vi "TDMSCreateGraph.vi"(8 "error in (no error)":errorcluster, 9 "States":string, 10 "FitModel":string, 11 "TraceName":string="D:\\Vi\\Data\\Singapore\\170620\\data_145.tdms: 3") -> (0 "error out":errorcluster, 2 "F(z) Graph":cluster{"Data":dbl[], "Data":dbl[]}[](graph), 3 "z(t) Graph":cluster{"Data":dbl[], "Data":dbl[]}[](graph))   [LabVIEW 2018]
uses:
  <vilib>/Analysis/polynomials.llb/Unique Numbers and Multiplicity (DBL).vi
  <vilib>/Analysis/NI_AALPro.lvlib
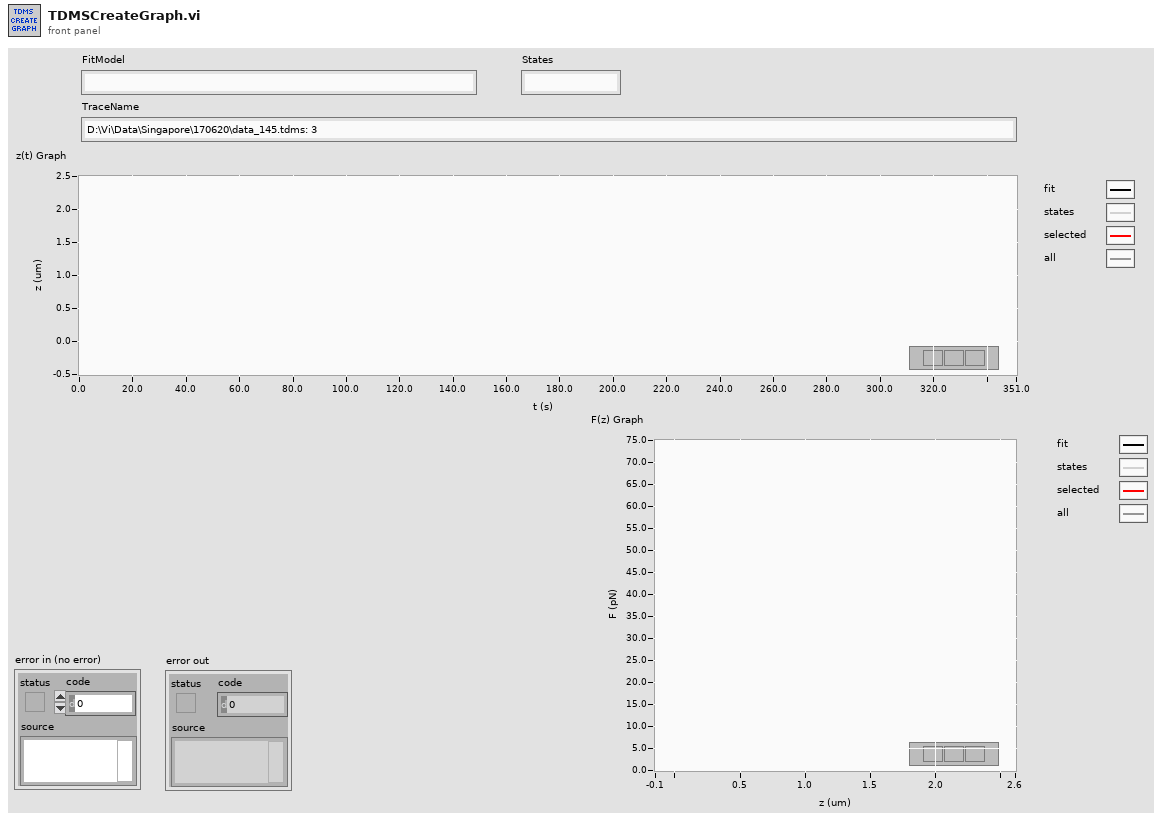
[diagram p1: front panel]
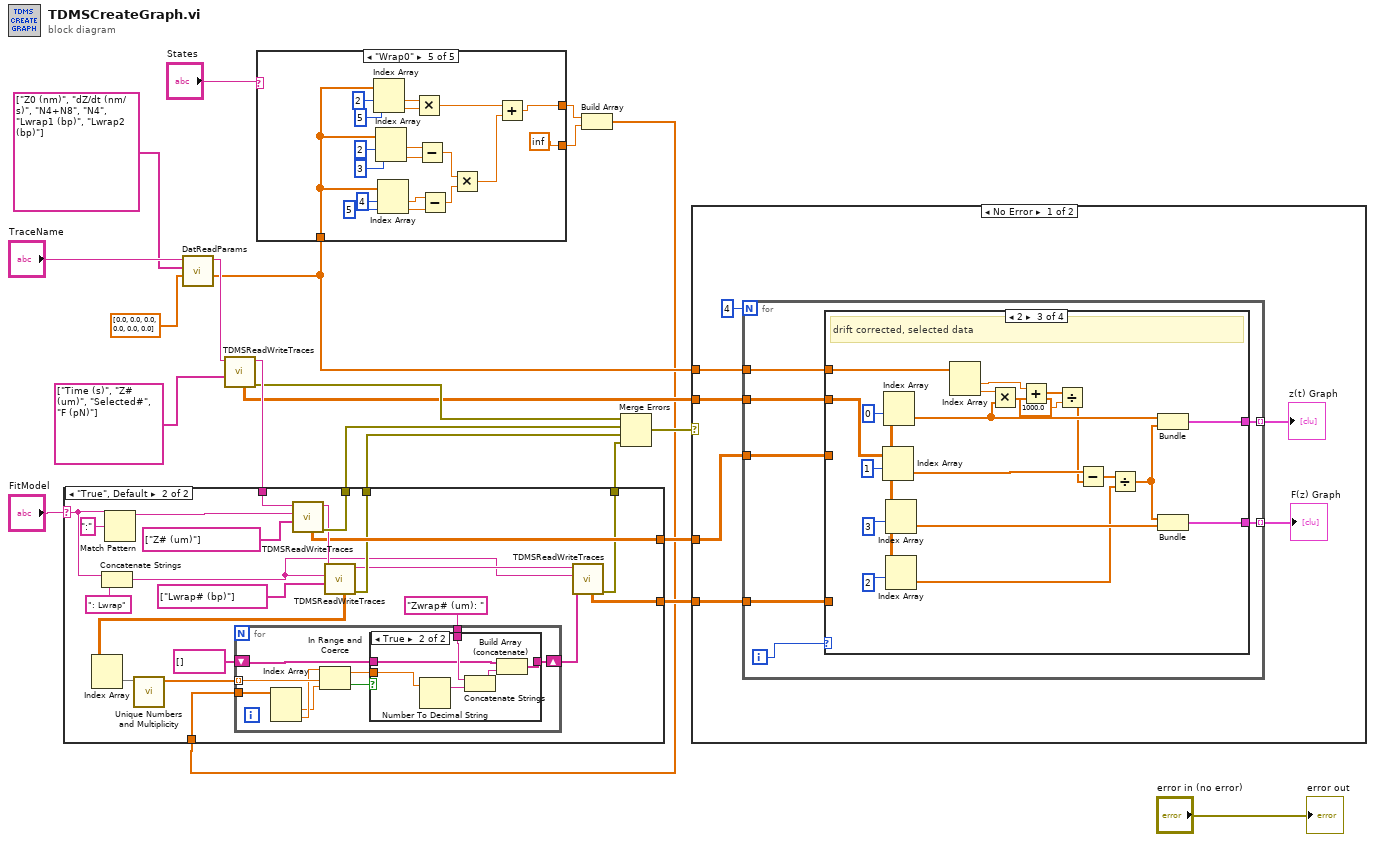
[diagram p0: block diagram]
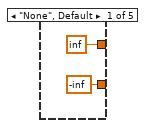
[diagram p2: hidden frame]
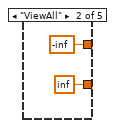
[diagram p3: hidden frame]
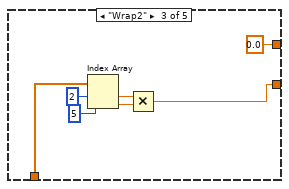
[diagram p4: hidden frame]
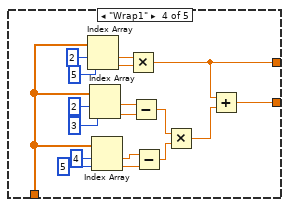
[diagram p5: hidden frame]
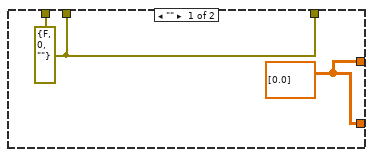
[diagram p6: hidden frame]
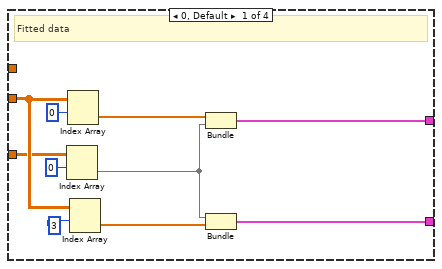
[diagram p8: hidden frame]
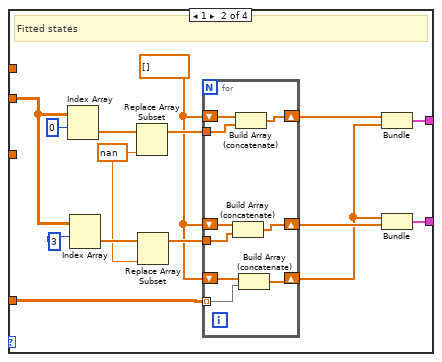
[diagram p9: hidden frame]
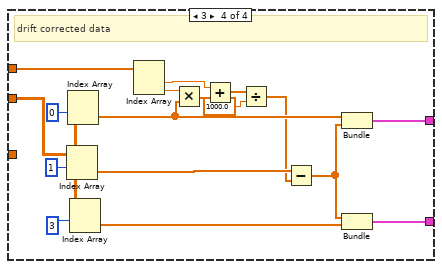
[diagram p10: hidden frame]
diagram:
  n1 = call "DatReadParams.vi"("default Values"=dbl[] [0.0, 0.0, 0.0, 0.0, 0.0, 0.0] ("Default values"), "Names"=string[] ["Z0 (nm)", "dZ/dt (nm/s)", "N4+N8", "N4", "Lwrap1 (bp)", "Lwrap2 (bp)"] ("Par names"), "tracename"="TraceName") -> ("Values out"=w2:dbl[], "tracename out"=w16:string)  [unwired: 4 in, 1 out]
  n2 = call "TDMSReadWriteTraces.vi"("Channels in"=string[] ["Time (s)", "Z# (um)", "Selected#", "F (pN)"] ("channel name(s) in"), "tracename"=w16) -> ("error out"=w15:errorcluster, "tracename out"=w20:string, "Data out"=w7:dbl[][])  [unwired: 4 in, 3 out]
  n3 = case shown="\"Wrap0\"" "States" {
    tunnel: [inf -inf 0.0 w34 w52] -> w4
    tunnel: [-inf inf w27 w33 inf] -> w3
    tunnel: w2 -> [_ _ w32 w42 w61]
    frame "None", Default {
    }
    frame "ViewAll" {
    }
    frame "Wrap2" {
      n4 = Index Array(array=w32, index #1=2 ("index"), index #2=5 ("index")) -> (element #1=w28:dbl, element #2=w29:dbl)
      n5 = Multiply(x=w28, y=w29) -> (x*y=w27:dbl)
    }
    frame "Wrap1" {
      n6 = Index Array(array=w42, index #1=2 ("index"), index #2=5 ("index")) -> (element #1=w47:dbl, element #2=w48:dbl)
      n7 = Index Array(array=w42, index #1=2 ("index"), index #2=3 ("index")) -> (element #1=w44:dbl, element #2=w45:dbl)
      n8 = Index Array(array=w42, index #1=4 ("index"), index #2=5 ("index")) -> (element #1=w38:dbl, element #2=w39:dbl)
      n9 = Multiply(x=w47, y=w48) -> (x*y=w34:dbl)
      n10 = Subtract(x=w44, y=w45) -> (x-y=w36:dbl)
      n11 = Subtract(x=w38, y=w39) -> (x-y=w37:dbl)
      n12 = Multiply(x=w36, y=w37) -> (x*y=w35:dbl)
      n13 = Add(x=w34, y=w35) -> (x+y=w33:dbl)
    }
    frame "Wrap0" {
      n14 = Index Array(array=w61, index #1=2 ("index"), index #2=5 ("index")) -> (element #1=w66:dbl, element #2=w67:dbl)
      n15 = Index Array(array=w61, index #1=2 ("index"), index #2=3 ("index")) -> (element #1=w63:dbl, element #2=w64:dbl)
      n16 = Index Array(array=w61, index #1=4 ("index"), index #2=5 ("index")) -> (element #1=w57:dbl, element #2=w58:dbl)
      n17 = Multiply(x=w66, y=w67) -> (x*y=w53:dbl)
      n18 = Subtract(x=w63, y=w64) -> (x-y=w55:dbl)
      n19 = Subtract(x=w57, y=w58) -> (x-y=w56:dbl)
      n20 = Multiply(x=w55, y=w56) -> (x*y=w54:dbl)
      n21 = Add(x=w53, y=w54) -> (x+y=w52:dbl)
    }
  }
  n22 = Build Array(w4, w3) -> (w1:dbl[])
  n23 = case shown="\"True\", Default" "FitModel" {
    selector: "FitModel" -> [_ w77]
    tunnel: w20 -> [_ w92]
    tunnel: [w71 w91] -> w14
    tunnel: [w70 w87] -> w12
    tunnel: [w71 w86] -> w11
    tunnel: [w71 w81] -> w9
    tunnel: [w70 w80] -> w8
    tunnel: w1 -> [_ w76]
    frame "" {
      w70 = dbl[][] [[0.0]] ("Data out")
      w71 = errorcluster {"status"=FALSE, "code"=0, "source"=""} ("error out")
    }
    frame "True", Default {
      n24 = Concatenate Strings(w77, ": Lwrap" ("string")) -> (w79:string)
      n25 = Match Pattern(string=w77, regular expression=":") -> (before substring=w88:string)  [unwired: 1 in, 3 out]
      n26 = call "TDMSReadWriteTraces.vi"("Channels in"=string[] ["Z# (um)"] ("channel name(s) in"), "group name"=w88, "tracename"=w92) -> ("error out"=w91:errorcluster, "tracename out"=w90:string, "Data out"=w87:dbl[][])  [unwired: 3 in, 3 out]
      n27 = call "TDMSReadWriteTraces.vi"("Channels in"=string[] ["Lwrap# (bp)"], "group name"=w79, "tracename"=w90) -> ("error out"=w86:errorcluster, "tracename out"=w82:string, "Data out"=w84:dbl[][])  [unwired: 3 in, 3 out]
      n28 = Index Array(array=w84) -> (element=w83:dbl[])  [unwired: 2 in]
      n29 = call-poly <vilib>:"Unique Numbers and Multiplicity.vi"("Numbers"=w83) -> ("Unique Numbers"=w75:dbl[])  [unwired: 8 in, 2 out]
      n30 = for {
        shift-right: [w96] -> w73
        shift-left: string[] [] -> [w95]
        tunnel: w76 -> [w102]
        tunnel: w75 -> [w101] mode=indexing
        tunnel: "Zwrap# (um): " ("Channel name") -> [w97]
        n31 = Index Array(array=w102) -> (element #1=w99:dbl, element #2=w100:dbl)  [unwired: 2 in]
        n32 = In Range and Coerce(upper limit=w100, x=w101, lower limit=w99) -> (coerced(x)=w94:dbl, In Range?=w98:bool)
        n33 = case shown="True" w98 {
          tunnel: w97 -> [_ w108]
          tunnel: [w103 w107] -> w96
          tunnel: w95 -> [w103 w105]
          tunnel: w94 -> [_ w104]
          frame False {
          }
          frame True {
            n34 = Number To Decimal String(number=w104) -> (decimal integer string=w109:string)  [unwired: 1 in]
            n35 = Concatenate Strings(w108, w109) -> (w106:string)
            n36 = Build Array (concatenate)(w105, w106) -> (w107:string[])
          }
        }
      }
      n37 = call "TDMSReadWriteTraces.vi"("Channels in"=w73, "group name"=w79, "tracename"=w82) -> ("error out"=w81:errorcluster, "Data out"=w80:dbl[][])  [unwired: 3 in, 4 out]
    }
  }
  n38 = Merge Errors(w15, w14, w11, w9) -> (w10:errorcluster)
  n39 = case shown="No Error" w10 {
    tunnel: w7 -> [w115 _]
    tunnel: w12 -> [w114 _]
    tunnel: w8 -> [w113 _]
    tunnel: w2 -> [w110 _]
    frame No Error {
      n40 = for {
        N: 4 -> [_]
        tunnel: w110 -> [w122]
        tunnel: w115 -> [w121]
        tunnel: [w120] -> w112 mode=indexing
        tunnel: [w119] -> w111 mode=indexing
        tunnel: w114 -> [w118]
        tunnel: w113 -> [w117]
        i -> [w123]
        n41 = case shown="2" w123 {
          tunnel: w122 -> [_ _ w170 w185]
          tunnel: w121 -> [w129 w146 w161 w190]
          tunnel: [w127 w145 w172 w187] -> w120
          tunnel: [w125 w144 w171 w186] -> w119
          tunnel: w118 -> [w126 _ _ _]
          tunnel: w117 -> [_ w136 _ _]
          frame 0, Default {
            # "Fitted data"
            n42 = Index Array(array=w126, index (row)=0) -> (element=w124:dbl[])  [unwired: 1 in]
            n43 = Index Array(array=w129, index (row)=0) -> (element=w131:dbl[])  [unwired: 1 in]
            n44 = Index Array(array=w129, index (row)=3) -> (element=w128:dbl[])  [unwired: 1 in]
            n45 = Bundle("Data out"=w131, "Data out"=w124) -> (w127:cluster{"Data out":dbl[], "Data out":dbl[]})  [unwired: 1 in]
            n46 = Bundle("Data out"=w124, "Data out"=w128) -> (w125:cluster{"Data out":dbl[], "Data out":dbl[]})  [unwired: 1 in]
          }
          frame 1 {
            w135 = dbl[] []
            w141 = nan ("new element/subarray")
            # "Fitted states"
            n47 = Index Array(array=w146, index (row)=0) -> (element=w143:dbl[])  [unwired: 1 in]
            n48 = Index Array(array=w146, index (row)=3) -> (element=w142:dbl[])  [unwired: 1 in]
            n49 = Replace Array Subset(array=w143, new element=w141) -> (w140:dbl[])  [unwired: 1 in]
            n50 = Replace Array Subset(array=w142, new element=w141) -> (w139:dbl[])  [unwired: 1 in]
            n51 = for {
              shift-right: [w155] -> w137
              shift-left: w135 -> [w157]
              shift-right: [w153] -> w138
              shift-left: w135 -> [w154]
              tunnel: w140 -> [w156]
              tunnel: w139 -> [w152]
              tunnel: w136 -> [w149] mode=indexing
              shift-right: [w151] -> w134
              shift-left: w135 -> [w150]
              n52 = Build Array (concatenate)(w154, w152) -> (w153:dbl[])
              n53 = Build Array (concatenate)(w157, w156) -> (w155:dbl[])
              n54 = Build Array (concatenate)(w150, w149) -> (w151:dbl[])
            }
            n55 = Bundle(w137, w134) -> (w145:cluster{dbl[], dbl[]})  [unwired: 1 in]
            n56 = Bundle(w134, w138) -> (w144:cluster{dbl[], dbl[]})  [unwired: 1 in]
          }
          frame 2 {
            # "drift corrected, selected data"
            n57 = Index Array(array=w161, index (row)=1) -> (element=w176:dbl[])  [unwired: 1 in]
            n58 = Index Array(array=w161, index (row)=0) -> (element=w168:dbl[])  [unwired: 1 in]
            n59 = Index Array(array=w161, index (row)=3) -> (element=w173:dbl[])  [unwired: 1 in]
            n60 = Index Array(array=w161, index (row)=2) -> (element=w158:dbl[])  [unwired: 1 in]
            n61 = Index Array(array=w170) -> (element #1=w166:dbl, element #2=w169:dbl)  [unwired: 2 in]
            n62 = Multiply(x=w169, y=w168) -> (x*y=w167:dbl[])
            n63 = Add(x=w166, y=w167) -> (x+y=w165:dbl[])
            n64 = Divide(x=w165, y=1000.0 ("element")) -> (x/y=w163:dbl[])
            n65 = Subtract(x=w176, y=w163) -> (x-y=w160:dbl[])
            n66 = Divide(x=w160, y=w158) -> (x/y=w159:dbl[])
            n67 = Bundle("Data out"=w168, w159) -> (w172:cluster{"Data out":dbl[], dbl[]})  [unwired: 1 in]
            n68 = Bundle(w159, "Data out"=w173) -> (w171:cluster{dbl[], "Data out":dbl[]})  [unwired: 1 in]
          }
          frame 3 {
            # "drift corrected data"
            n69 = Index Array(array=w190, index (row)=1) -> (element=w193:dbl[])  [unwired: 1 in]
            n70 = Index Array(array=w190, index (row)=0) -> (element=w183:dbl[])  [unwired: 1 in]
            n71 = Index Array(array=w190, index (row)=3) -> (element=w189:dbl[])  [unwired: 1 in]
            n72 = Index Array(array=w185) -> (element #1=w181:dbl, element #2=w184:dbl)  [unwired: 2 in]
            n73 = Multiply(x=w184, y=w183) -> (x*y=w182:dbl[])
            n74 = Add(x=w181, y=w182) -> (x+y=w180:dbl[])
            n75 = Divide(x=w180, y=1000.0 ("element")) -> (x/y=w178:dbl[])
            n76 = Subtract(x=w193, y=w178) -> (x-y=w188:dbl[])
            n77 = Bundle("Data out"=w183, w188) -> (w187:cluster{"Data out":dbl[], dbl[]})  [unwired: 1 in]
            n78 = Bundle(w188, "Data out"=w189) -> (w186:cluster{dbl[], "Data out":dbl[]})  [unwired: 1 in]
          }
        }
      }
      "z(t) Graph" <- w112
      "F(z) Graph" <- w111
    }
    frame Error {
    }
  }
  "error out" <- "error in (no error)"
